vi "Save Settings to XML.vi"(8 "error in (no error)":errorcluster, 11 "Settings":T1) -> (0 "error out":errorcluster)   [LabVIEW 2018, in "Settings.lvlib"]
doc: "Saves the \"User Specified\" configuration data to an XML file. This is used to remember the users settings between executions."
uses:
  Settings.lvlib
  Settings.ctl
  Acquisition/Hardware Configuration.ctl
  Logging/Logging Configuration.ctl
  controls/UI RefNums.ctl
  <vilib>/Utility/xml.llb/Write to XML File(string).vi
  Acquisition/Acquisition.lvlib
  Logging/Logging.lvlib
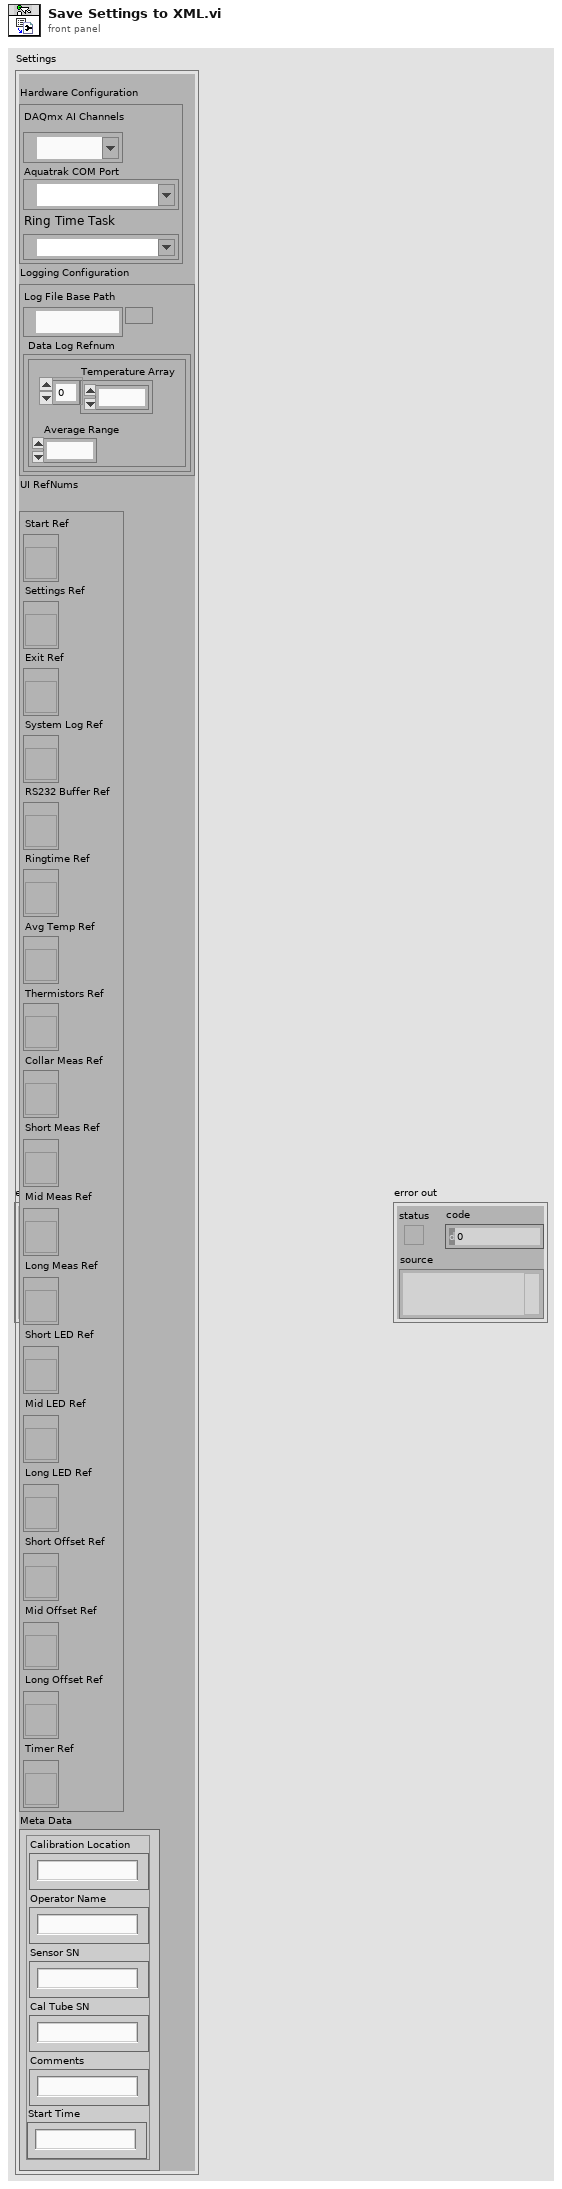
[diagram p1: front panel]
types:
  T1 = typedef "Settings.ctl" = cluster{"Hardware Configuration":T2, "Logging Configuration":T3, "UI RefNums":T4, "Meta Data":cluster{"Calibration Location":string, "Operator Name":string, "Sensor SN":string, "Cal Tube SN":string, "Comments":string, "Start Time":string}}
  T2 = typedef "Acquisition.lvlib/Hardware Configuration.ctl" = cluster{"DAQmx AI Channels":tag, "Aquatrak COM Port":refnum<visa-resource-name>, "Ring Time Task":refnum<k21>}
  T3 = typedef "Logging.lvlib/Logging Configuration.ctl" = cluster{"Log File Base Path":path, "Data Log Refnum":refnum<k1>}
  T4 = typedef "UI RefNums.ctl" = cluster{"Start Ref":refnum<vi>, "Settings Ref":refnum<vi>, "Exit Ref":refnum<vi>, "System Log Ref":refnum<vi>, "RS232 Buffer Ref":refnum<vi>, "Ringtime Ref":refnum<vi>, "Avg Temp Ref":refnum<vi>, "Thermistors Ref":refnum<vi>, "Collar Meas Ref":refnum<vi>, "Short Meas Ref":refnum<vi>, "Mid Meas Ref":refnum<vi>, "Long Meas Ref":refnum<vi>, "Short LED Ref":refnum<vi>, "Mid LED Ref":refnum<vi>, "Long LED Ref":refnum<vi>, "Short Offset Ref":refnum<vi>, "Mid Offset Ref":refnum<vi>, "Long Offset Ref":refnum<vi>, "Timer Ref":refnum<vi>}
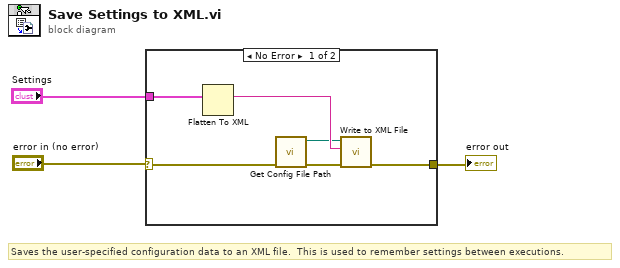
[diagram p0: block diagram]
diagram:
  # "Saves the user-specified configuration data to an XML file.  This is used to remember settings between executions."
  n1 = case shown="No Error" "error in (no error)" {
    selector: "error in (no error)" -> [w5 w10]
    tunnel: [w7 w10] -> w2
    tunnel: "Settings" -> [w9 _]
    frame No Error {
      n2 = Flatten To XML(anything=w9) -> (xml string=w8:string)
      n3 = call "Get Config File Path.vi"("error in (no error)"=w5) -> ("error out"=w4:errorcluster, "XML File Path"=w6:path)  [unwired: 9 in]
      n4 = call-poly <vilib>:"Write to XML File.vi"("error in (no error)"=w4, "XML Input"=w8, "XML File Path"=w6) -> ("error out"=w7:errorcluster)  [unwired: 6 in, 2 out]
    }
    frame Error {
    }
  }
  "error out" <- w2
